vi "Completa_2_caractere.vi"(2 "Carac para Completar":string, 3 "entrada":string) -> (1 "saida":string)   [LabVIEW 2012]
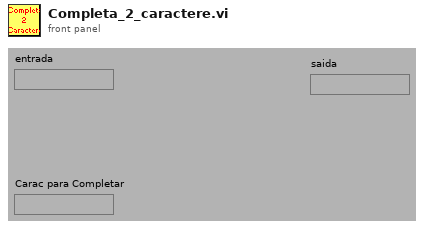
[diagram p1: front panel]
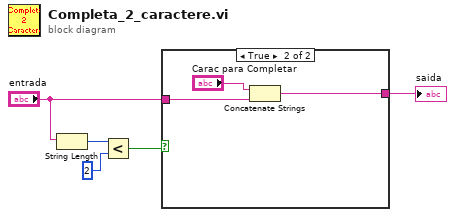
[diagram p0: block diagram]
diagram:
  n1 = String Length(string="entrada") -> (length=w1:i32)
  n2 = Less?(x=w1, y=2) -> (x < y?=w3:bool)
  n3 = case shown="True" w3 {
    tunnel: "entrada" -> [w6 w9]
    tunnel: [w6 w8] -> w5
    frame False {
    }
    frame True {
      n4 = Concatenate Strings("Carac para Completar", w9) -> (w8:string)
    }
  }
  "saida" <- w5
